vi "Subscribe Request.vi"(6 "Broadcaster":string, 8 "error in (no error)":errorcluster, 9 "Subscriber Enqueuer":refnum<class "Message Enqueuer.lvclass">, 10 "Topic":string, 11 "Measure Object in":refnum<class "da Base.lvclass">) -> (0 "error out":errorcluster, 3 "Measure Object out":refnum<class "da Base.lvclass">)   [LabVIEW 2016, in "da Base.lvclass"]
uses:
  da Base.lvclass
  <vilib>/ActorFramework/Message Enqueuer/Message Enqueuer.lvclass
  da Base.lvclass/da Base.ctl
  Da Base Messages/Subscribe Request Msg/Subscribe Request Msg.lvclass/Subscribe Request Msg.ctl
  <vilib>/ActorFramework/Message Enqueuer/Message Enqueuer.lvclass/Message Enqueuer.ctl
  Read Name.vi
  <vilib>/ActorFramework/Message Enqueuer/Enqueue.vi
  Da Base Messages/Subscribe Request Msg/Subscribe Request Msg.lvclass
  C:/Program Files/National Instruments/LabVIEW 2016/vi.lib/ActorFramework/Message/Message.lvclass
  <vilib>/ActorFramework/Message Priority Queue/Priority Enqueue.vi
  BroadcastBroker/BroadcastBroker.lvclass
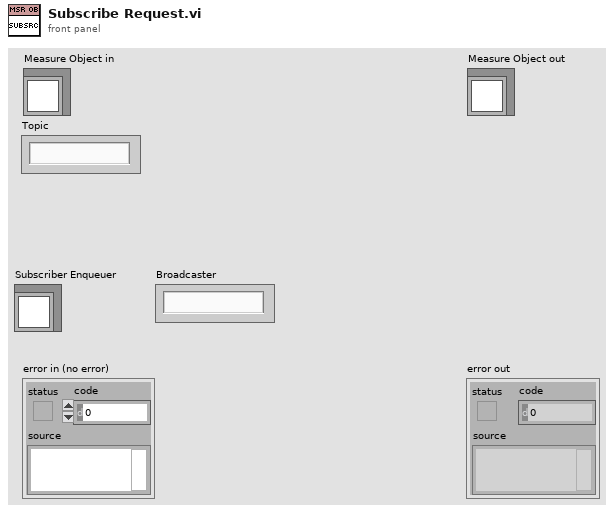
[diagram p1: front panel]
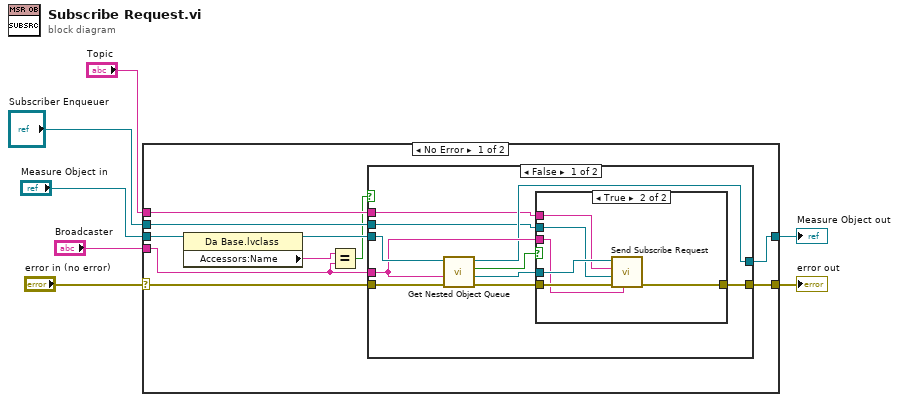
[diagram p0: block diagram]
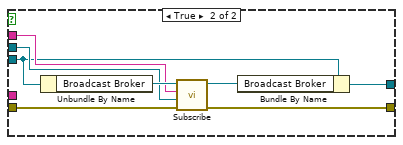
[diagram p3: hidden frame]
diagram:
  n1 = case shown="No Error" "error in (no error)" {
    selector: "error in (no error)" -> [w16 w44]
    tunnel: [w15 w44] -> w6
    tunnel: [w14 w43] -> w4
    tunnel: "Measure Object in" -> [w17 w43]
    tunnel: "Subscriber Enqueuer" -> [w13 _]
    tunnel: "Topic" -> [w12 _]
    tunnel: "Broadcaster" -> [w8 _]
    frame No Error {
      n2 = property class="Da Base.lvclass"(reference=w17) -> (reference out=w11:refnum<class "da Base.lvclass">, "Accessors:Name"=w10:string)  [unwired: 1 in, 1 out]
      n3 = Equal?(x=w10, y=w8) -> (x = y?=w9:bool)
      n4 = case shown="False" w9 {
        tunnel: w16 -> [w26 w41]
        tunnel: [w21 w40] -> w15
        tunnel: [w20 w39] -> w14
        tunnel: w13 -> [w19 w37]
        tunnel: w12 -> [w18 w36]
        tunnel: w11 -> [w27 w35]
        tunnel: w8 -> [w22 _]
        frame False {
          n5 = call-dynamic "Get Nested Object Queue.vi"("error in (no error)"=w26, "Name"=w22, "Measure Object in"=w27) -> ("error out"=w23:errorcluster, "Object Enqueuer"=w24:refnum<class "Message Enqueuer.lvclass">, "Found?"=w25:bool, "Measure Object out"=w20:refnum<class "da Base.lvclass">)  [unwired: 5 in]
          n6 = case shown="True" w25 {
            tunnel: w24 -> [_ w34]
            tunnel: w23 -> [w28 w33]
            tunnel: w22 -> [_ w32]
            tunnel: [w28 w31] -> w21
            tunnel: w19 -> [_ w30]
            tunnel: w18 -> [_ w29]
            frame False {
            }
            frame True {
              n7 = call "Send Subscribe Request.vi"("Broadcaster"=w32, "error in (no error)"=w33, "Subscriber Enqueuer"=w30, "Topic"=w29, "Message Enqueuer"=w34) -> ("error out"=w31:errorcluster)  [unwired: 5 in, 1 out]
            }
          }
        }
        frame True {
          n8 = Unbundle By Name(w35) -> ("Broadcast Broker"=w42:refnum<class "BroadcastBroker.lvclass">)
          n9 = call-dynamic "Subscribe.vi"("error in (no error)"=w41, "Subscriber Enqueuer"=w37, "Topic"=w36, "Broadcaster in"=w42) -> ("error out"=w40:errorcluster, "Broadcaster out"=w38:refnum<class "BroadcastBroker.lvclass">)  [unwired: 6 in]
          n10 = Bundle By Name(cluster=w35, "Broadcast Broker"=w38) -> (w39:refnum<class "da Base.lvclass">)
        }
      }
    }
    frame Error {
    }
  }
  "error out" <- w6
  "Measure Object out" <- w4
